vi "Initialise.vi"(8 "error in (no error)":errorcluster, 11 "Time to wait":dbl) -> (0 "error out":errorcluster, 3 "StopInstruction out":refnum<class "StopInstruction.lvclass">)   [LabVIEW 2015, in "StopInstruction.lvclass"]
uses:
  StopInstruction.lvclass
  StopInstruction.lvclass/StopInstruction.ctl
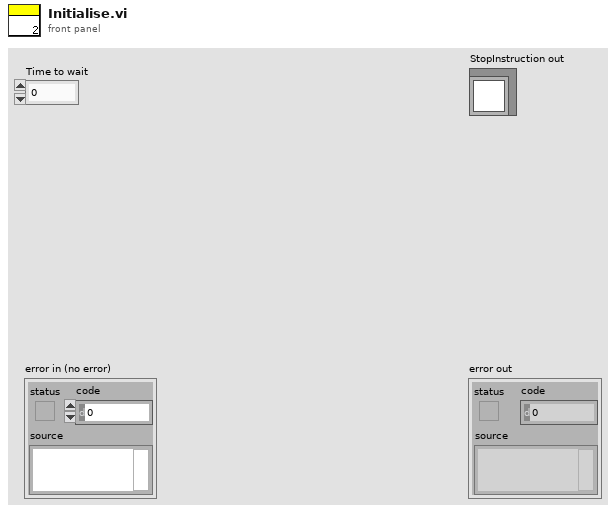
[diagram p1: front panel]
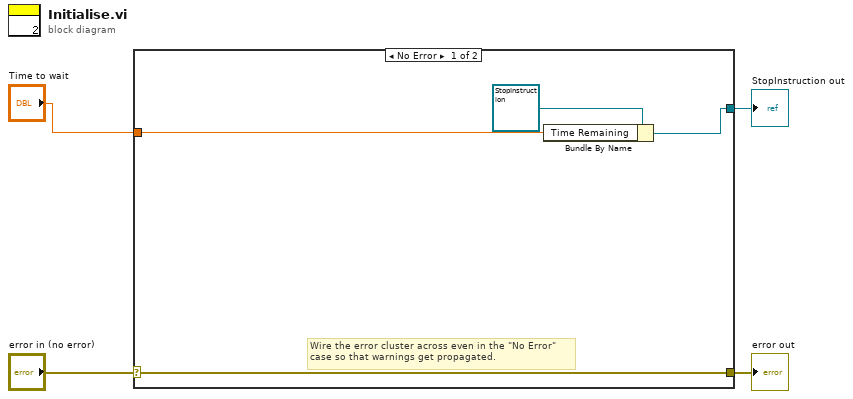
[diagram p0: block diagram]
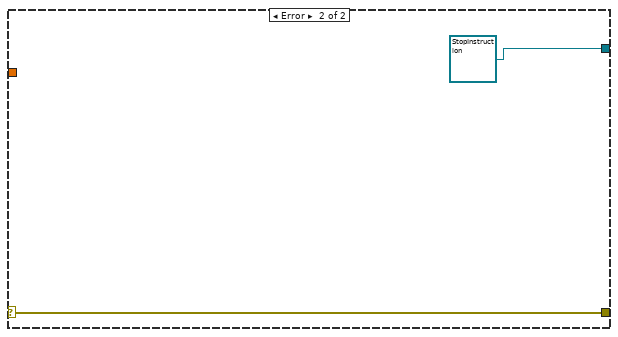
[diagram p2: hidden frame]
diagram:
  n1 = case shown="No Error" "error in (no error)" {
    selector: "error in (no error)" -> [w8 w10]
    tunnel: [w8 w10] -> w3
    tunnel: [w5 refnum<class "StopInstruction.lvclass"> refnum ("StopInstruction.lvclass")] -> w2
    tunnel: "Time to wait" -> [w6 _]
    frame No Error {
      # "Wire the error cluster across even in the \"No Error\"\ncase so that warnings get propagated."
      n2 = Bundle By Name(cluster=refnum<class "StopInstruction.lvclass"> refnum ("StopInstruction.lvclass"), "Time Remaining"=w6) -> (w5:refnum<class "StopInstruction.lvclass">)
    }
    frame Error {
    }
  }
  "error out" <- w3
  "StopInstruction out" <- w2
